vi "6221_write_waveform_debug_standalone.vi"(6 "Error In":errorcluster, 7 "Counter Task In":refnum<k21>, 8 "Waveform Task In":refnum<k21>, 9 "ODT Params":T1={"Waveform Parameters"=[[{"Initial Value"=0.0, "Final Value"=0.0, "Tau"=0.0, "Eta"=0.0, "Nickname"="Channel 0 A", "Enum"=enum."Power Law"}, {"Initial Value"=0.0, "Final Value"=0.0, "Tau"=0.0, "Eta"=0.0, "Nickname"="Channel 0 B", "Enum"=enum."Power Law"}, {"Initial Value"=0.0, "Final Value"=0.0, "Tau"=0.0, "Eta"=0.0, "Nickname"="Channel 0 C", "Enum"=enum."Power Law"}, {"Initial Value"=0.0, "Final Value"=0.0, "Tau"=0.0, "Eta"=0.0, "Nickname"="Channel 0 D", "Enum"=enum."Power Law"}], [{"Initial Value"=0.0, "Final Value"=0.0, "Tau"=0.0, "Eta"=0.0, "Nickname"="Channel 1 A", "Enum"=enum."Power Law"}, {"Initial Value"=0.0, "Final Value"=0.0, "Tau"=0.0, "Eta"=0.0, "Nickname"="Channel 1 B", "Enum"=enum."Power Law"}, {"Initial Value"=0.0, "Final Value"=0.0, "Tau"=0.0, "Eta"=0.0, "Nickname"="Channel 1 C", "Enum"=enum."Power Law"}, {"Initial Value"=0.0, "Final Value"=0.0, "Tau"=0.0, "Eta"=0.0, "Nickname"="Channel 1 D", "Enum"=enum."Power Law"}]], "Active Phases"=[TRUE, FALSE, FALSE, FALSE], "Active Channels"=[FALSE, FALSE], "Phase Times (s)"=[0.001, 0.0, 0.0, 0.0], "Active Device"="6221_ODT", "Trigger Channel"="/6221_ODT/PFI0"} {"Phase Times (s)" format="%#_6p"}) -> (0 "Error Out":errorcluster, 1 "Counter Task Out":refnum<k21>, 2 "Waveform Task Out":refnum<k21>)   [LabVIEW 2013]
uses:
  6221_panel.ctl
  6221_waveform_param.ctl
  6221_states.ctl
  <vilib>/DAQmx/write.llb/DAQmx Write (Analog 1D DBL NChan 1Samp).vi
  <vilib>/DAQmx/write.llb/DAQmx Write (Analog 1D Wfm NChan NSamp).vi
  <vilib>/DAQmx/create/channels.llb/DAQmx Create Channel (AO-Voltage-Basic).vi
  <vilib>/DAQmx/miscellaneous.llb/DAQmx Fill In Error Info.vi
  <vilib>/Waveform/WDTOps.llb/WDT Append Waveforms DBL.vi
  <vilib>/DAQmx/configure/timing.llb/DAQmx Timing (Sample Clock).vi
  <vilib>/DAQmx/create/channels.llb/DAQmx Create Channel (CO-Pulse Generation-Frequency).vi
  <vilib>/DAQmx/configure/timing.llb/DAQmx Timing (Implicit).vi
  <vilib>/DAQmx/configure/trigger.llb/DAQmx Start Trigger (Digital Edge).vi
  <vilib>/Waveform/WDTOps.llb/WDT Scale Delta t DBL.vi
  <resource>/objmgr/daqmx.rc
panel:
  out "element":waveform(dbl)(graph)
  in  "index":i32
  out "Samples Written":dbl
  out "Waveforms":waveform(dbl)[](array[waveform])
  out "Sample Rate":dbl
  out "Max Sample Rate":dbl
  out "Total Time":dbl
  out "Inactive Channels":tag[](array[tag])
  out "Active Channels":tag[](array[tag])
  out "# Inactive Channels":i32
  out "# Active Channels":i32
  out "AO.Voltage.Rngs":dbl[](array[numeric])
  out "AO.PhysicalChans":tag[](array[tag])
  out "Active Device":tag
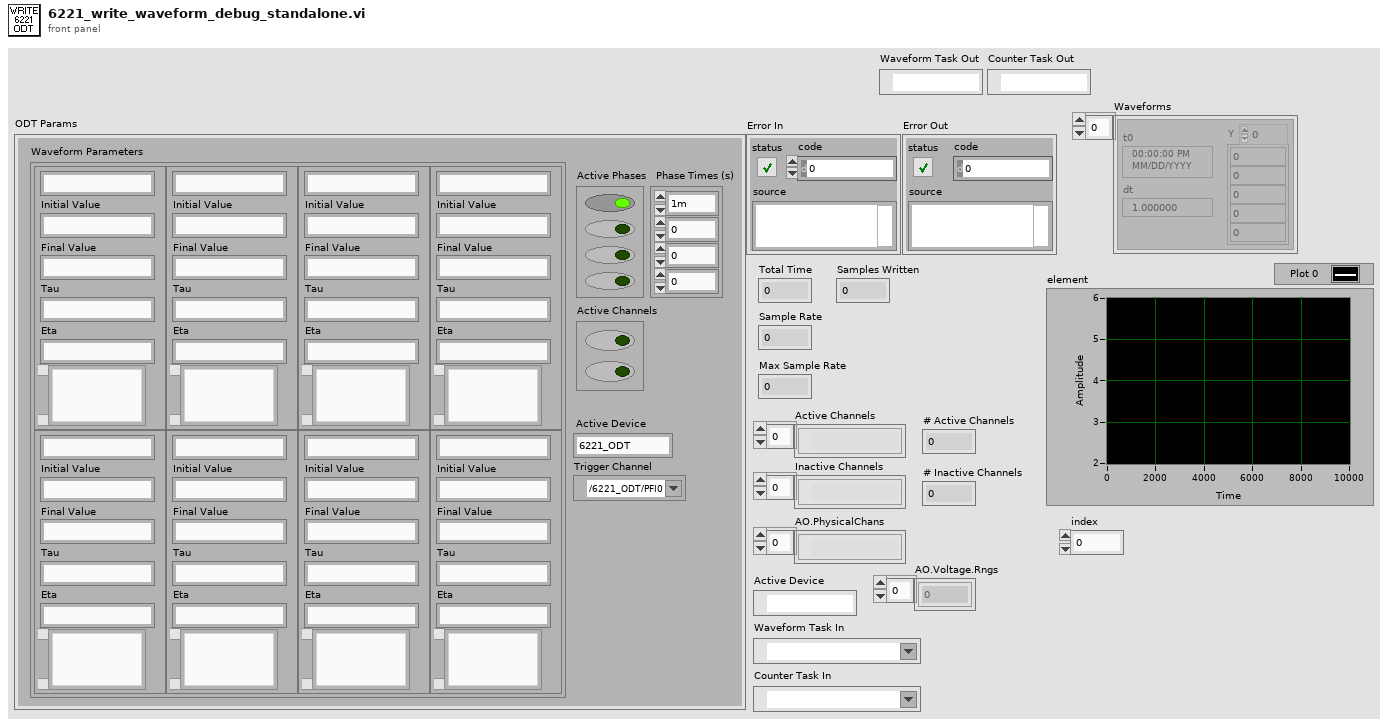
[diagram p1: front panel]
types:
  T1 = typedef "6221_panel.ctl" = cluster{"Waveform Parameters":T2[][], "Active Phases":bool[], "Active Channels":bool[], "Phase Times (s)":dbl[], "Active Device":string, "Trigger Channel":tag}
  T2 = typedef "6221_waveform_param.ctl" = cluster{"Initial Value":dbl, "Final Value":dbl, "Tau":dbl, "Eta":dbl, "Nickname":string, "Enum":enum16{"Volts to Volts", "Power Law", "Evaporation Formula"}}
  T3 = typedef "6221_states.ctl" = enum16{"Write to Cards", "Check for Problems", "Write Waveforms", "Maximize Samples / Channel", "Clear Old Tasks", "Get Active/Inactive Channels", "Get Device Information", "Initialize"}
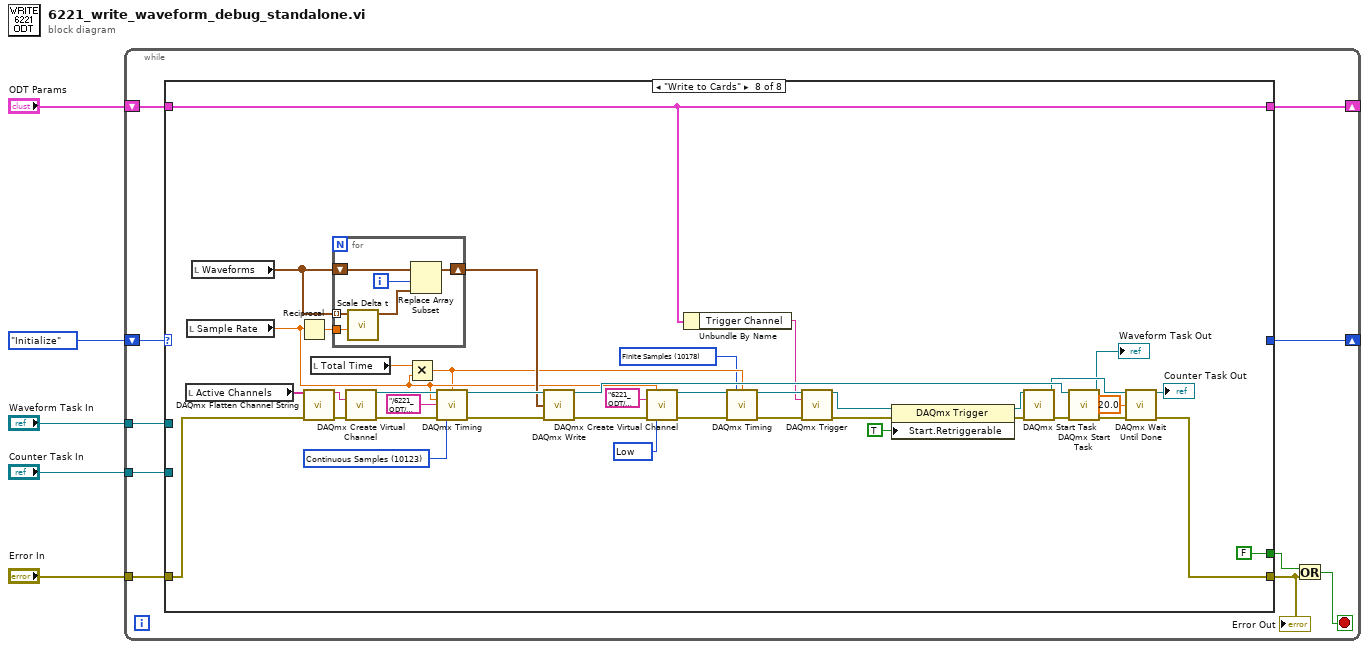
[diagram p0: block diagram]
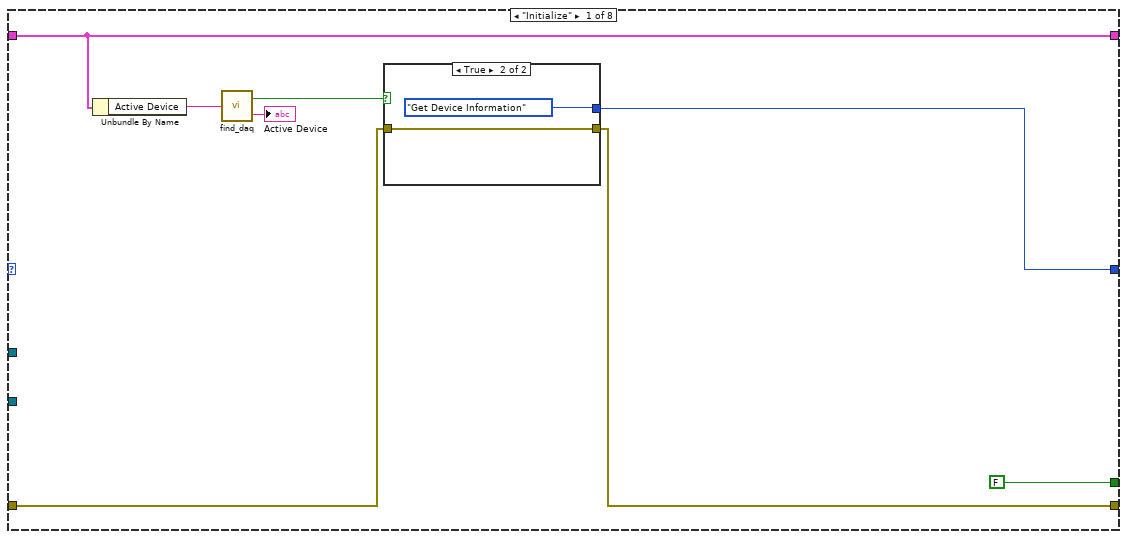
[diagram p2: hidden frame]
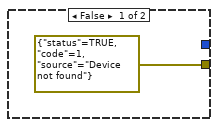
[diagram p3: hidden frame]
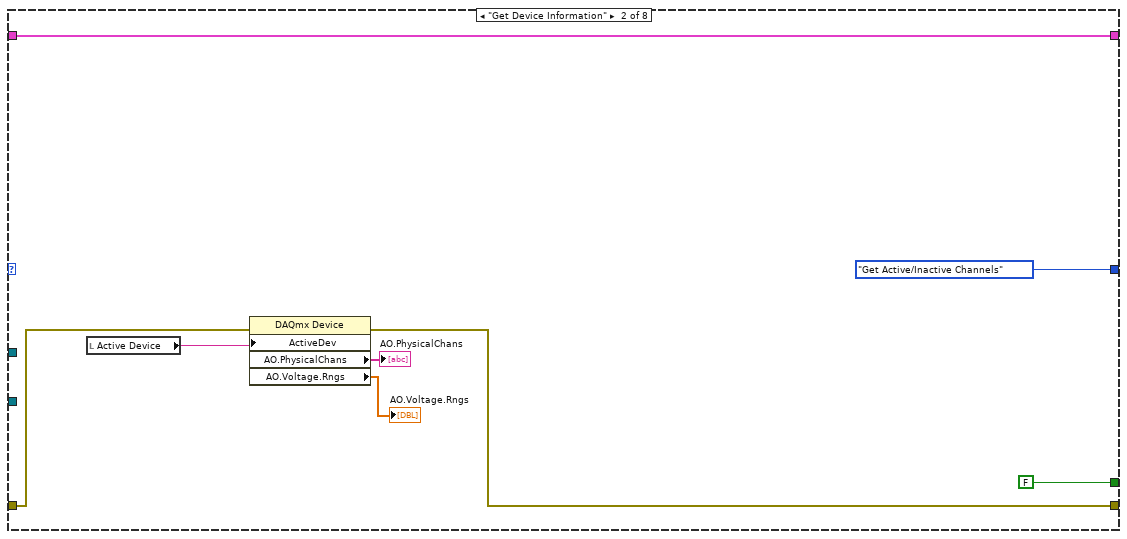
[diagram p4: hidden frame]
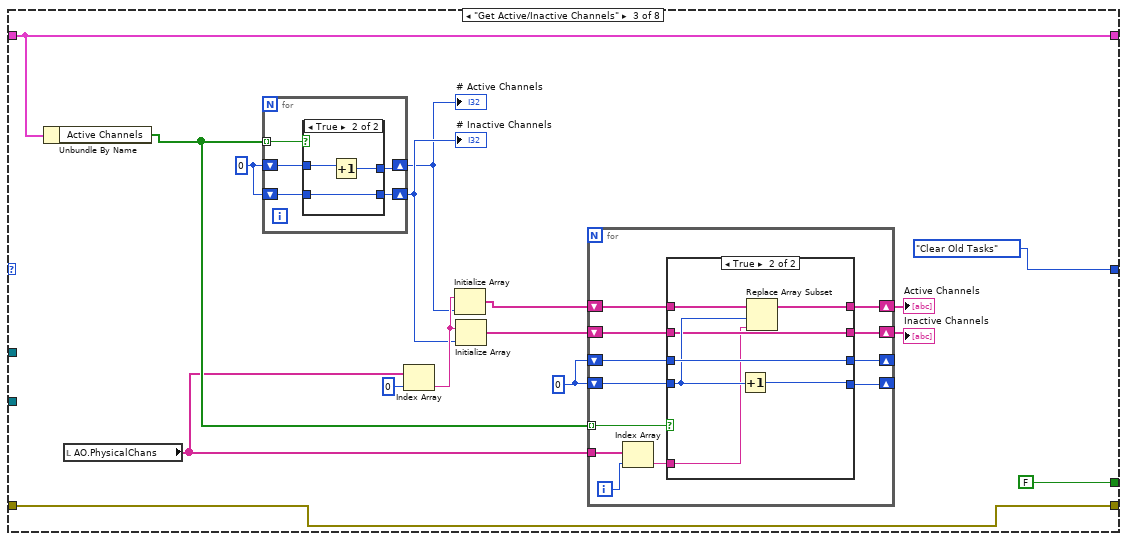
[diagram p5: hidden frame]
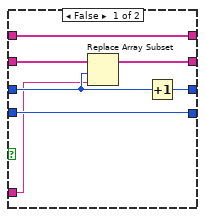
[diagram p6: hidden frame]
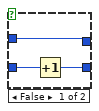
[diagram p7: hidden frame]
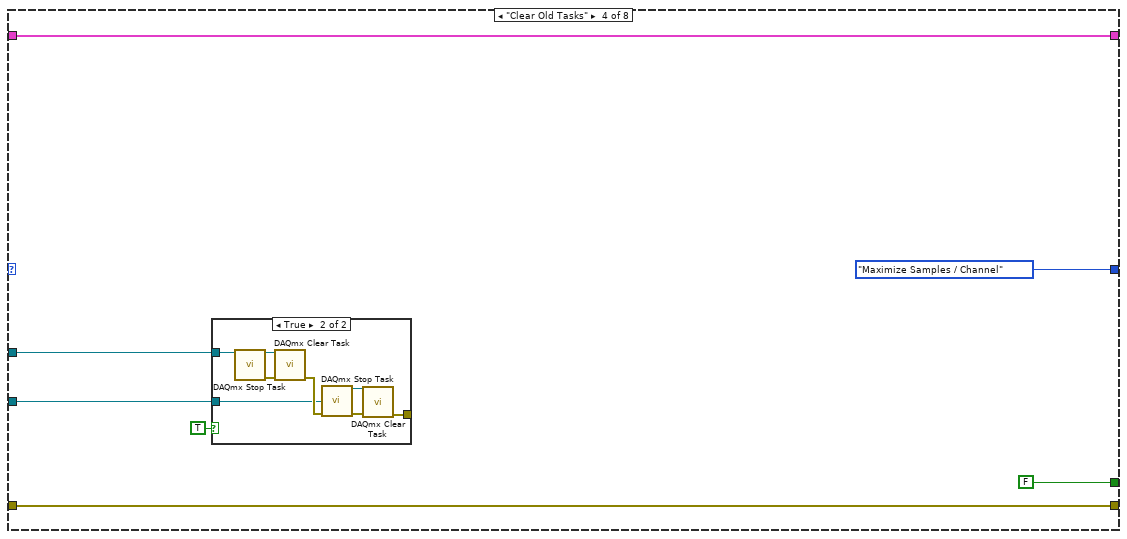
[diagram p8: hidden frame]
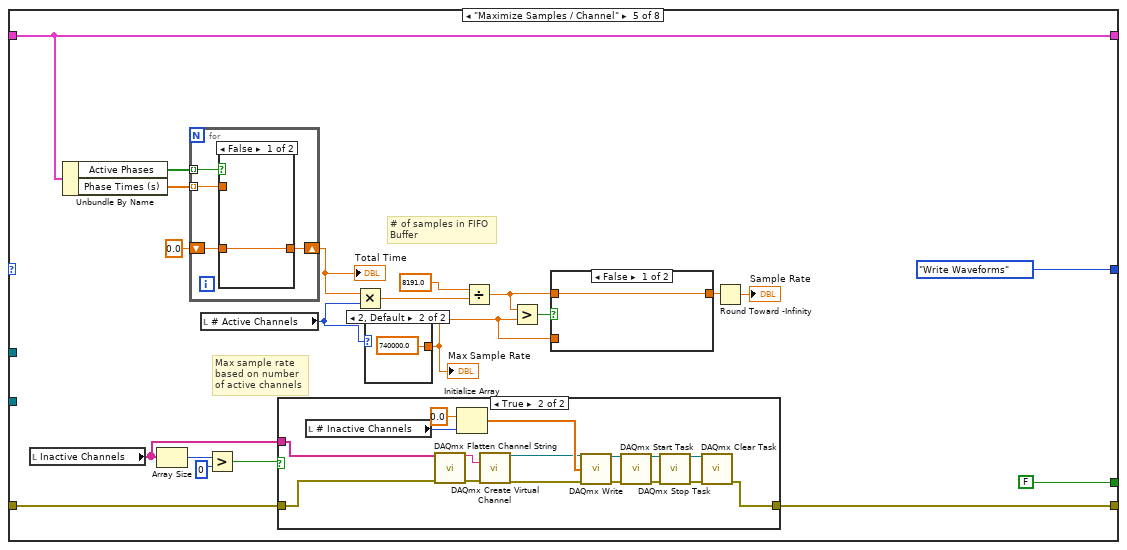
[diagram p10: hidden frame]
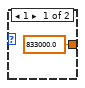
[diagram p13: hidden frame]
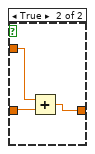
[diagram p14: hidden frame]
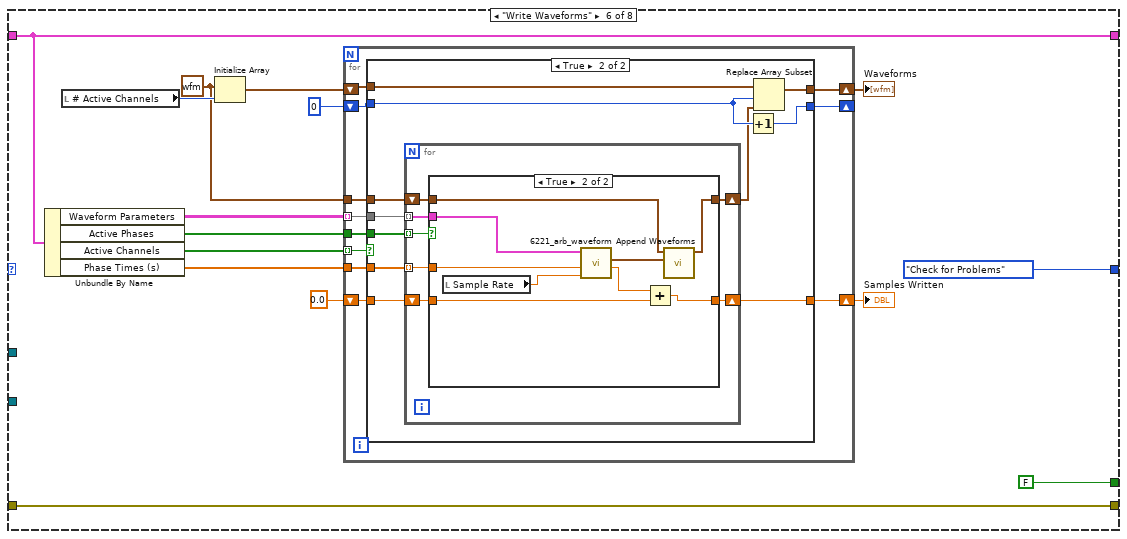
[diagram p15: hidden frame]
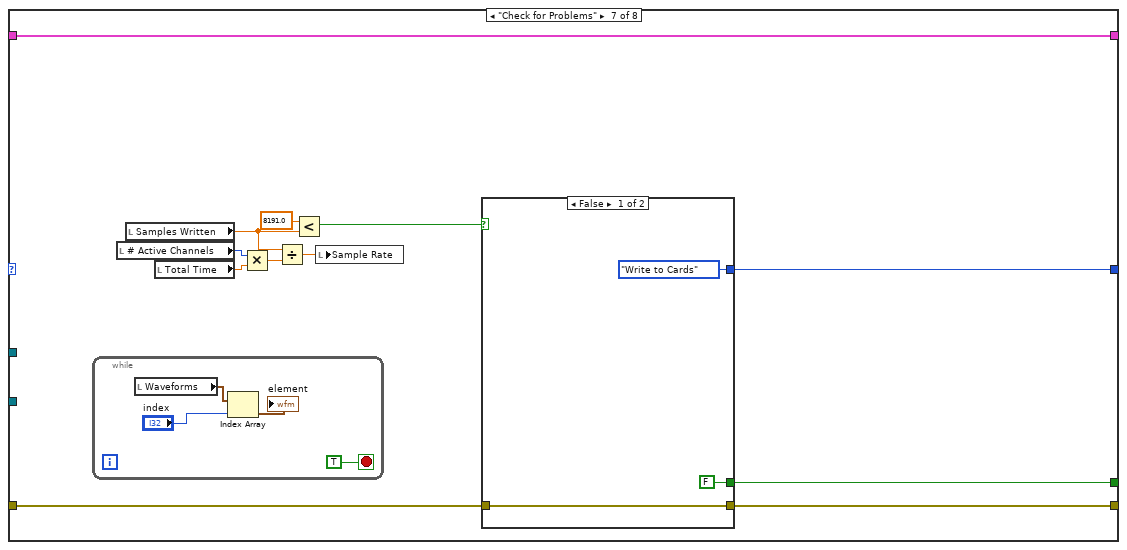
[diagram p18: hidden frame]
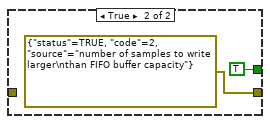
[diagram p19: hidden frame]
diagram:
  n1 = while {
    shift-right: [w12] -> _
    shift-left: 6221_states."Initialize" -> [w15]
    shift-right: [w13] -> _
    shift-left: "ODT Params" -> [w14]
    tunnel: "Error In" -> [w11]
    tunnel: "Waveform Task In" -> [w7]
    tunnel: "Counter Task In" -> [w6]
    stop <- w9 stop-if-true
    n2 = case shown="\"Write to Cards\"" w15 {
      tunnel: w14 -> [w23 w30 w50 w94 w120 w165 w222 w242]
      tunnel: [w23 w30 w50 w94 w120 w165 w222 w242] -> w13
      tunnel: [w19 6221_states."Get Active/Inactive Channels" 6221_states."Clear Old Tasks" 6221_states."Maximize Samples / Channel" 6221_states."Write Waveforms" 6221_states."Check for Problems" w214 _] -> w12
      tunnel: w11 -> [w18 w33 w48 w90 w123 w167 w211 w269]
      tunnel: [w17 w29 w48 w90 w122 w167 w212 w236] -> w8
      tunnel: [FALSE FALSE FALSE FALSE FALSE FALSE w213 FALSE] -> w10
      tunnel: w7 -> [_ _ _ w92 _ _ _ _]
      tunnel: w6 -> [_ _ _ w91 _ _ _ _]
      frame "Initialize" {
        n3 = Unbundle By Name(w23) -> ("Active Device"=w22:string)
        n4 = call "find_daq.vi"("Device Name"=w22) -> ("Device Present"=w20:bool, "DAQmx Device Name"=→"Active Device":tag)
        n5 = case shown="True" w20 {
          tunnel: [_ 6221_states."Get Device Information"] -> w19
          tunnel: w18 -> [_ w25]
          tunnel: [errorcluster {"status"=TRUE, "code"=1, "source"="Device not found"} ("Error In") w25] -> w17
          frame False {
          }
          frame True {
          }
        }
      }
      frame "Get Device Information" {
        n6 = local read "Active Device"() -> (w34:tag)
        n7 = property class="DAQmx Device"(error in=w33, "ActiveDev"=w34) -> (error out=w29:errorcluster, "AO.PhysicalChans"=→"AO.PhysicalChans":tag[], "AO.Voltage.Rngs"=→"AO.Voltage.Rngs":dbl[])  [unwired: 1 in, 1 out]
      }
      frame "Get Active/Inactive Channels" {
        w41 = 0
        w35 = 0
        n8 = Unbundle By Name(w50) -> ("Active Channels"=w47:bool[])
        n9 = local read "AO.PhysicalChans"() -> (w46:tag[])
        n10 = for {
          tunnel: w47 -> [w81] mode=indexing
          shift-right: [w77] -> w43
          shift-left: w35 -> [w80]
          shift-right: [w78] -> w42
          shift-left: w35 -> [w79]
          n11 = case shown="True" w81 {
            tunnel: w80 -> [w82 w85]
            tunnel: w79 -> [w84 w87]
            tunnel: [w84 w86] -> w78
            tunnel: [w83 w85] -> w77
            frame False {
              n12 = Increment(x=w82) -> (x+1=w83:i32)
            }
            frame True {
              n13 = Increment(x=w87) -> (x+1=w86:i32)
            }
          }
        }
        "# Active Channels" <- w42
        "# Inactive Channels" <- w43
        n14 = Index Array(array=w46, index=0) -> (element=w44:tag)
        n15 = Initialize Array(w44, w42) -> (w39:tag[])
        n16 = Initialize Array(w44, w43) -> (w40:tag[])
        n17 = for {
          tunnel: w47 -> [w62] mode=indexing
          tunnel: w46 -> [w60]
          shift-right: [w51] -> w37
          shift-left: w40 -> [w52]
          shift-right: [w54] -> w38
          shift-left: w39 -> [w55]
          shift-right: [w56] -> _
          shift-left: w41 -> [w58]
          shift-right: [w53] -> _
          shift-left: w41 -> [w57]
          i -> [w61]
          n18 = Index Array(array=w60, index=w61) -> (element=w59:tag)
          n19 = case shown="True" w62 {
            tunnel: w59 -> [w63 w70]
            tunnel: w58 -> [w69 w73]
            tunnel: w57 -> [w66 w74]
            tunnel: [w69 w72] -> w56
            tunnel: w55 -> [w67 w76]
            tunnel: [w67 w75] -> w54
            tunnel: [w68 w74] -> w53
            tunnel: w52 -> [w65 w71]
            tunnel: [w64 w71] -> w51
            frame False {
              n20 = Replace Array Subset(array=w65, new element=w63, index=w66) -> (w64:tag[])
              n21 = Increment(x=w66) -> (x+1=w68:i32)
            }
            frame True {
              n22 = Increment(x=w73) -> (x+1=w72:i32)
              n23 = Replace Array Subset(array=w76, new element=w70, index=w73) -> (w75:tag[])
            }
          }
        }
        "Active Channels" <- w38
        "Inactive Channels" <- w37
      }
      frame "Clear Old Tasks" {
        n24 = case shown="True" TRUE {
          tunnel: [_ w97] -> _
          tunnel: w92 -> [_ w96]
          tunnel: w91 -> [_ w95]
          frame False {
          }
          frame True {
            n25 = call <vilib>:"DAQmx Stop Task.vi"("task/channels in"=w96) -> ("task out"=w101:refnum<k21>, "error out"=w102:errorcluster)  [unwired: 13 in]
            n26 = call <vilib>:"DAQmx Clear Task.vi"("task in"=w101, "error in"=w102) -> ("error out"=w98:errorcluster)  [unwired: 13 in]
            n27 = call <vilib>:"DAQmx Stop Task.vi"("task/channels in"=w95, "error in"=w98) -> ("task out"=w100:refnum<k21>, "error out"=w99:errorcluster)  [unwired: 12 in]
            n28 = call <vilib>:"DAQmx Clear Task.vi"("task in"=w100, "error in"=w99) -> ("error out"=w97:errorcluster)  [unwired: 13 in]
          }
        }
      }
      frame "Maximize Samples / Channel" {
        # "Max sample rate\nbased on number\nof active channels"
        # "# of samples in FIFO\nBuffer"
        n29 = local read "Inactive Channels"() -> (w103:tag[])
        n30 = Unbundle By Name(w120) -> ("Active Phases"=w118:bool[], "Phase Times (s)"=w119:dbl[])
        n31 = Array Size(array=w103) -> (size(s)=w106:i32)
        n32 = for {
          tunnel: w119 -> [w147] mode=indexing
          tunnel: w118 -> [w148] mode=indexing
          shift-right: [w145] -> w116
          shift-left: 0.0 -> [w146]
          n33 = case shown="False" w148 {
            tunnel: w147 -> [_ w150]
            tunnel: w146 -> [w149 w152]
            tunnel: [w149 w151] -> w145
            frame False {
            }
            frame True {
              n34 = Add(x=w150, y=w152) -> (x+y=w151:dbl)
            }
          }
        }
        "Total Time" <- w116
        n35 = local read "# Active Channels"() -> (w113:i32)
        n36 = Greater?(x=w106, y=0) -> (0:w104:bool)
        n37 = case shown="True" w104 {
          tunnel: w123 -> [w124 w140]
          tunnel: [w124 w126] -> w122
          tunnel: w103 -> [_ w125]
          frame False {
          }
          frame True {
            n38 = local read "# Inactive Channels"() -> (w135:i32)
            n39 = call <vilib>:"DAQmx Flatten Channel String.vi"("names in"=w125, "error in"=w140) -> ("names out"=w138:string, "error out"=w139:errorcluster)  [unwired: 12 in]
            n40 = Initialize Array(0.0 ("element"), w135) -> (w134:dbl[])
            n41 = call-poly <vilib>:"DAQmx Create Virtual Channel.vi"("physical channels"=w138, "error in"=w139) -> ("task out"=w133:refnum<k21>, "error out"=w137:errorcluster)  [unwired: 12 in]
            n42 = call-poly <vilib>:"DAQmx Write.vi"("task/channels in"=w133, "data"=w134, "error in"=w137) -> ("task out"=w132:refnum<k21>, "error out"=w131:errorcluster)  [unwired: 10 in, 1 out]
            n43 = call <vilib>:"DAQmx Start Task.vi"("task/channels in"=w132, "error in"=w131) -> ("task out"=w130:refnum<k21>, "error out"=w129:errorcluster)  [unwired: 12 in]
            n44 = call <vilib>:"DAQmx Stop Task.vi"("task/channels in"=w130, "error in"=w129) -> ("task out"=w128:refnum<k21>, "error out"=w127:errorcluster)  [unwired: 12 in]
            n45 = call <vilib>:"DAQmx Clear Task.vi"("task in"=w128, "error in"=w127) -> ("error out"=w126:errorcluster)  [unwired: 13 in]
          }
        }
        n46 = Multiply(x=w116, y=w113) -> (x*y=w115:dbl)
        n47 = case shown="2, Default" w113 {
          tunnel: [833000.0 740000.0] -> w110
          frame 1 {
          }
          frame 2, Default {
          }
        }
        "Max Sample Rate" <- w110
        n48 = Divide(x=8191.0, y=w115) -> (x/y=w111:dbl)
        n49 = Greater?(x=w111, y=w110) -> (0:w112:bool)
        n50 = case shown="False" w112 {
          tunnel: w111 -> [w141 _]
          tunnel: w110 -> [_ w142]
          tunnel: [w141 w142] -> w109
          frame False {
          }
          frame True {
          }
        }
        n51 = Round Toward -Infinity(1:w109) -> (0:→"Sample Rate":dbl)
      }
      frame "Write Waveforms" {
        w154 = waveform(dbl) {"t0"=timestamp(0 s since 1904-01-01), "dt"=1.0, "Y"=[]} ("waveform")
        n52 = Unbundle By Name(w165) -> ("Waveform Parameters"=w157:T2[][], "Active Phases"=w159:bool[], "Active Channels"=w160:bool[], "Phase Times (s)"=w158:dbl[])
        n53 = local read "# Active Channels"() -> (w164:i32)
        n54 = Initialize Array(w154, w164) -> (w163:waveform(dbl)[])
        n55 = for {
          shift-right: [w176] -> w161
          shift-left: w163 -> [w175]
          shift-right: [w177] -> _
          shift-left: 0 -> [w174]
          tunnel: w160 -> [w178] mode=indexing
          tunnel: w159 -> [w173]
          tunnel: w158 -> [w172]
          tunnel: w157 -> [w171] mode=indexing
          shift-right: [w169] -> w153
          shift-left: 0.0 ("y") -> [w170]
          tunnel: w154 -> [w168]
          n56 = case shown="True" w178 {
            tunnel: [w180 w192] -> w177
            tunnel: [w179 w191] -> w176
            tunnel: w175 -> [w179 w190]
            tunnel: w174 -> [w180 w189]
            tunnel: w173 -> [_ w188]
            tunnel: w172 -> [_ w187]
            tunnel: w171 -> [_ w186]
            tunnel: w170 -> [w181 w185]
            tunnel: [w181 w184] -> w169
            tunnel: w168 -> [_ w183]
            frame False {
            }
            frame True {
              n57 = for {
                tunnel: w188 -> [w199] mode=indexing
                tunnel: w187 -> [w197] mode=indexing
                tunnel: w186 -> [w198] mode=indexing
                shift-right: [w195] -> w184
                shift-left: w185 -> [w196]
                shift-right: [w193] -> w182
                shift-left: w183 -> [w194]
                n58 = case shown="True" w199 {
                  tunnel: w198 -> [_ w210]
                  tunnel: w197 -> [_ w209]
                  tunnel: w196 -> [w200 w206]
                  tunnel: [w200 w205] -> w195
                  tunnel: w194 -> [w201 w203]
                  tunnel: [w201 w202] -> w193
                  frame False {
                  }
                  frame True {
                    n59 = local read "Sample Rate"() -> (w208:dbl)
                    n60 = call "6221_arb_waveform.vi"("Waveform Input"=w210, "Phase Time"=w209, "Sample Rate"=w208) -> ("output waveform"=w204:waveform(dbl), "# Samples"=w207:dbl)  [unwired: 6 in]
                    n61 = Add(x=w207, y=w206) -> (x+y=w205:dbl)
                    n62 = call-poly <vilib>:"Append Waveforms.vi"("waveform B"=w204, "waveform A"=w203) -> ("waveform out"=w202:waveform(dbl))  [unwired: 8 in, 1 out]
                  }
                }
              }
              n63 = Increment(x=w189) -> (x+1=w192:i32)
              n64 = Replace Array Subset(array=w190, new element=w182, index=w189) -> (w191:waveform(dbl)[])
            }
          }
        }
        "Waveforms" <- w161
        "Samples Written" <- w153
      }
      frame "Check for Problems" {
        n65 = while {
          stop <- TRUE stop-if-true
          n66 = local read "Waveforms"() -> (w224:waveform(dbl)[])
          n67 = Index Array(array=w224, index="index") -> (element=→"element":waveform(dbl))
        }
        n68 = local read "# Active Channels"() -> (w219:i32)
        n69 = local read "Samples Written"() -> (w217:dbl)
        n70 = local read "Total Time"() -> (w220:dbl)
        n71 = Multiply(x=w219, y=w220) -> (x*y=w218:dbl)
        n72 = Divide(x=w217, y=w218) -> (x/y=w216:dbl)
        n73 = Less?(x=8191.0, y=w217) -> (x < y?=w215:bool)
        n74 = local write "Sample Rate"(w216) -> ()
        n75 = case shown="False" w215 {
          tunnel: [6221_states."Write to Cards" _] -> w214
          tunnel: [FALSE TRUE] -> w213
          tunnel: [w227 errorcluster {"status"=TRUE, "code"=2, "source"="number of samples to write larger\nthan FIFO buffer capacity"} ("error in (no error)")] -> w212
          tunnel: w211 -> [w227 _]
          frame False {
          }
          frame True {
          }
        }
      }
      frame "Write to Cards" {
        w238 = 10123 items=["Finite Samples"=10178, "Continuous Samples"=10123, "Hardware Timed Single Point"=12522] ("sample mode")
        w239 = 10214 items=["High"=10192, "Low"=10214] ("idle state")
        w240 = 10178 items=["Finite Samples"=10178, "Continuous Samples"=10123, "Hardware Timed Single Point"=12522] ("sample mode")
        n76 = local read "Active Channels"() -> (w270:tag[])
        n77 = local read "Sample Rate"() -> (w244:dbl)
        n78 = local read "Waveforms"() -> (w248:waveform(dbl)[])
        n79 = Reciprocal(x=w244) -> (1/x=w247:dbl)
        n80 = call <vilib>:"DAQmx Flatten Channel String.vi"("names in"=w270, "error in"=w269) -> ("names out"=w268:string, "error out"=w267:errorcluster)  [unwired: 12 in]
        n81 = local read "Total Time"() -> (w245:dbl)
        n82 = for {
          tunnel: w248 -> [w273] mode=indexing
          shift-right: [w276] -> w246
          shift-left: w248 -> [w277]
          tunnel: w247 -> [w274]
          i -> [w275]
          n83 = call-poly <vilib>:"Scale Delta t.vi"("scale factor"=w274, "waveform in"=w273) -> ("waveform out"=w272:waveform(dbl))  [unwired: 8 in, 1 out]
          n84 = Replace Array Subset(array=w277, new element=w272, index=w275) -> (w276:waveform(dbl)[])
        }
        n85 = call-poly <vilib>:"DAQmx Create Virtual Channel.vi"("physical channels"=w268, "error in"=w267) -> ("task out"=w264:refnum<k21>, "error out"=w266:errorcluster)  [unwired: 12 in]
        n86 = Multiply(x=w245, y=w244) -> (x*y=w243:dbl)
        n87 = call-poly <vilib>:"DAQmx Timing.vi"("task/channels in"=w264, "sample mode"=w238, "samples per channel"=w243, "rate"=w244, "source"=tag "/6221_ODT/Ctr0InternalOutput", "error in"=w266) -> ("task out"=w262:refnum<k21>, "error out"=w263:errorcluster)  [unwired: 8 in]
        n88 = call-poly <vilib>:"DAQmx Write.vi"("task/channels in"=w262, "data"=w246, "error in"=w263) -> ("task out"=w249:refnum<k21>, "error out"=w261:errorcluster)  [unwired: 10 in, 1 out]
        n89 = call-poly <vilib>:"DAQmx Create Virtual Channel.vi"("frequency"=w244, "counter"=tag "6221_ODT/ctr0", "error in"=w261, "idle state"=w239) -> ("task out"=w258:refnum<k21>, "error out"=w259:errorcluster)  [unwired: 10 in]
        n90 = Unbundle By Name(w242) -> ("Trigger Channel"=w241:tag)
        n91 = call-poly <vilib>:"DAQmx Timing.vi"("task/channels in"=w258, "sample mode"=w240, "samples per channel"=w243, "error in"=w259) -> ("task out"=w256:refnum<k21>, "error out"=w257:errorcluster)  [unwired: 10 in]
        n92 = call-poly <vilib>:"DAQmx Trigger.vi"("task/channels in"=w256, "source"=w241, "error in"=w257) -> ("task out"=w253:refnum<k21>, "error out"=w255:errorcluster)  [unwired: 11 in]
        n93 = property class="DAQmx Trigger"(reference=w253, error in=w255, "Start.Retriggerable"=TRUE) -> (reference out=w252:refnum<k21>, error out=w251:errorcluster)
        n94 = call <vilib>:"DAQmx Start Task.vi"("task/channels in"=w252, "error in"=w251) -> ("task out"=w234:refnum<k21>, "error out"=w250:errorcluster)  [unwired: 12 in]
        n95 = call <vilib>:"DAQmx Start Task.vi"("task/channels in"=w249, "error in"=w250) -> ("task out"=→"Waveform Task Out":refnum<k21>, "error out"=w237:errorcluster)  [unwired: 12 in]
        n96 = call <vilib>:"DAQmx Wait Until Done.vi"("task/channels in"=w234, "timeout (sec)"=20.0, "error in"=w237) -> ("task out"=→"Counter Task Out":refnum<k21>, "error out"=w236:errorcluster)  [unwired: 11 in]
      }
    }
    "Error Out" <- w8
    n97 = Or(x=w10, y=w8) -> (x .or. y?=w9:bool)
  }
